vi "Write LabJack Configuration.vi"(8 "error in (no error)":errorcluster, 10 "Configuration":T1={"Scale"=nan, "Offset"=0.0}, 11 "LabJack Driver in":refnum<class "LabJack Driver.lvclass">) -> (0 "error out":errorcluster, 3 "LabJack Driver out":refnum<class "LabJack Driver.lvclass">)   [LabVIEW 2021, in "LabJack Driver.lvclass"]
uses:
  LabJack Driver.lvclass
  C:/GitHub/NHMFL_Core/Libraries/Instruments/Instrument Driver/Instrument Driver.lvclass
  LabJack Configuration.ctl
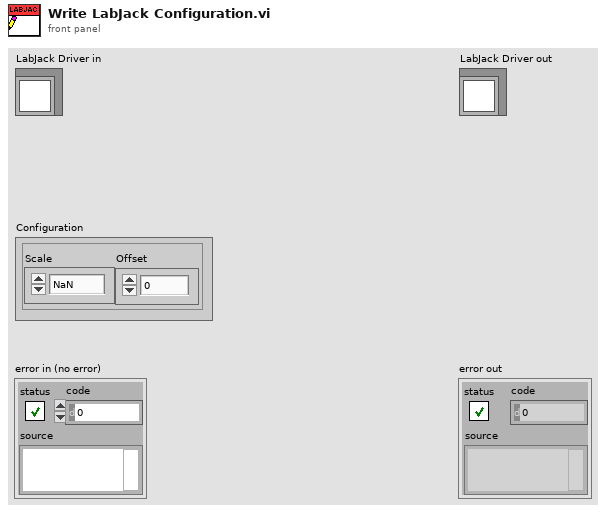
[diagram p1: front panel]
types:
  T1 = typedef "LabJack Configuration.ctl" = cluster{"Scale":dbl, "Offset":dbl}
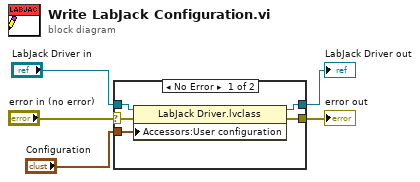
[diagram p0: block diagram]
diagram:
  n1 = case shown="No Error" "error in (no error)" {
    selector: "error in (no error)" -> [w7 w11]
    tunnel: [w6 w11] -> w4
    tunnel: [w10 w12] -> w2
    tunnel: "LabJack Driver in" -> [w9 w12]
    tunnel: "Configuration" -> [w8 _]
    frame No Error {
      n2 = property class="LabJack Driver.lvclass"(reference=w9, error in=w7, "Accessors:User configuration"=w8) -> (reference out=w10:refnum<class "LabJack Driver.lvclass">, error out=w6:errorcluster)
    }
    frame Error {
    }
  }
  "error out" <- w4
  "LabJack Driver out" <- w2
